vi "RFmx Analysis Only Configure Session.vi"(0 "IVI Refnum in":refnum<k15>="RFSA" caption="Resource Name", 1 "Span (Hz)":dbl=765000000.0 format="%.3p", 5 "Carrier Frequency (Hz)":dbl=4000000000.0 format="%#_6p", 7 "Reference Level (dBm)":dbl format="%.2f", 9 "number of records":i64=1, 11 "error in (no error)":errorcluster) -> (4 "RFSA Instrument Handle Out":refnum<k15>, 6 "RFmx Instrument Handle Out":T4, 15 "error out 2":errorcluster)   [LabVIEW 2017]
uses:
  <instrlib>/niRFSA/niRFSA.llb/niRFSA Ref Clock Sources.ctl
  <instrlib>/niRFSA/niRFSA.llb/niRFSA Exported Signal Destinations.ctl
  <instrlib>/niRFSA/niRFSA.llb/niRFSA Trigger Terminals.ctl
  <vilib>/RFmx/RFInstr/mx/Support/RFmxInstrSupport.llb/niRFmx Instrument Handle.ctl
  <instrlib>/niRFSA/niRFSA.llb/niRFSA Acquisition Types.ctl
  <instrlib>/niRFSA/niRFSA.llb/niRFSA Signal Names.ctl
  <vilib>/RFmx/SpecAn/mx/RFmxSpecAn.llb/RFmxSpecAn Select Measurement (Multiple).vi
  <instrlib>/niRFSA/niRFSA.llb/niRFSA Configure Digital Edge Start Trigger.vi
  <instrlib>/niRFSA/niRFSA.llb/niRFSA Configure Digital Edge Advance Trigger.vi
  <resource>/objmgr/RFmxInstr.rc
panel:
  in  "Integration Bandwidth (Hz)":dbl=5000000.0 format="%.3p"
  in  "source":T1="PXI_Trig0"
  in  "output terminal":T2="PXI_Trig1"
  in  "Clock Source":T3="OnboardClock"
  # "RFSA Settings"
  # "RFmx Settings"
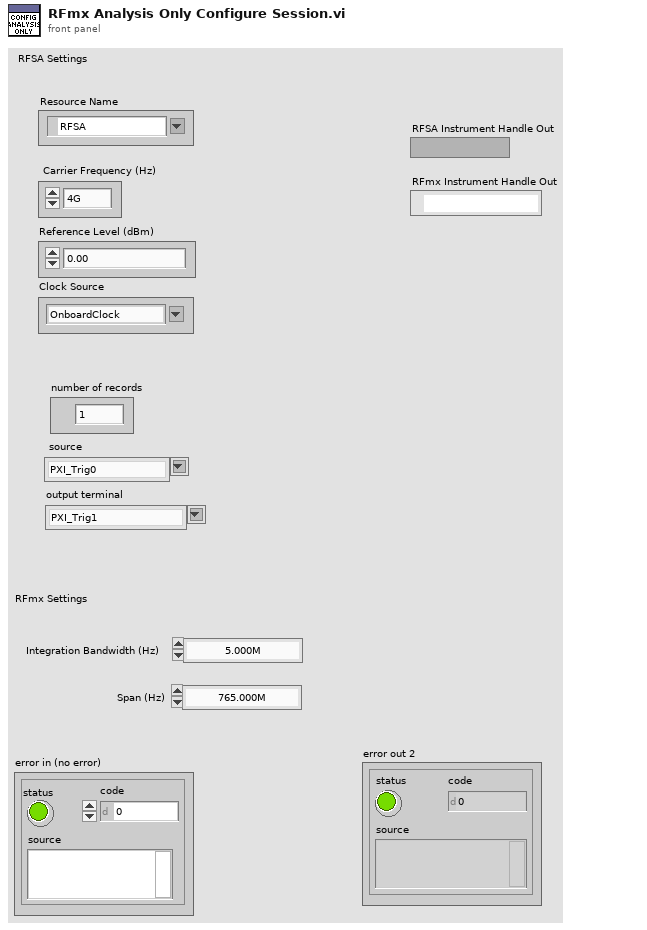
[diagram p1: front panel]
types:
  T1 = typedef "niRFSA Trigger Terminals.ctl" = string
  T2 = typedef "niRFSA Exported Signal Destinations.ctl" = string
  T3 = typedef "niRFSA Ref Clock Sources.ctl" = string
  T4 = typedef "niRFmx Instrument Handle.ctl" = refnum<k21>
  T5 = enum16{"ACP", "CCDF", "CHP", "FCnt", "Harmonics", "OBW", "SEM", "Spectrum", "Spur", "TXP", "AMPM", "DPD", "IQ", "IM", "NF", "PhaseNoise"}[]
  T6 = typedef "niRFSA Signal Names.ctl" = i32
  T7 = typedef "niRFSA Acquisition Types.ctl" = i32
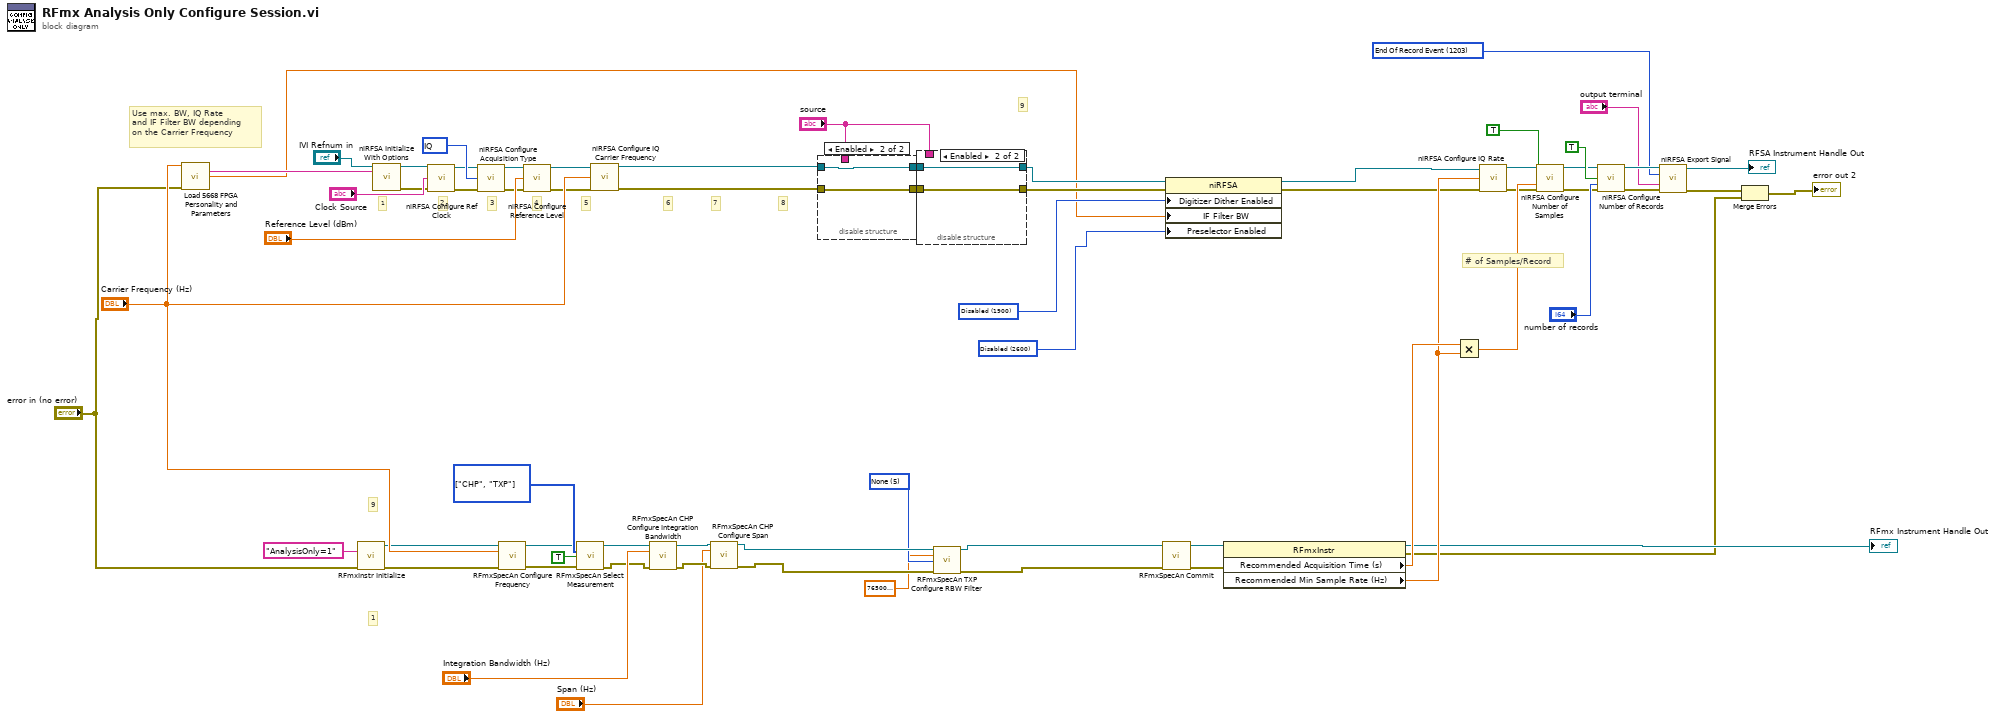
[diagram p0: block diagram]
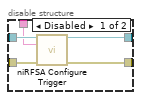
[diagram p2: hidden frame]
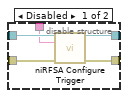
[diagram p3: hidden frame]
diagram:
  w3 = 5 items=["None"=5, "Gaussian"=1, "Flat"=2, "RRC"=6] ("RBW Filter Type")
  w67 = T5 [enum."CHP", enum."TXP"] items=["ACP", "CCDF", "CHP", "FCnt", "Harmonics", "OBW", "SEM", "Spectrum", "Spur", "TXP", "AMPM", "DPD", "IQ", "IM", "NF", "PhaseNoise"] ("Measurements")
  w45 = 2600 items=["Disabled"=2600, "Enabled when in Signal Path"=2601, "Enabled"=2602] ("Signal Path:Advanced:Downconverter Preselector Enabled")
  w44 = 1900 items=["Disabled"=1900, "Enabled"=1901] ("Signal Path:Digitizer Dither Enabled")
  w32 = T6 1203 items=["Start Trigger"=1100, "Ref Trigger"=702, "Advance Trigger"=1102, "Ready For Start Event"=1200, "Ready For Ref Event"=1201, "Ready For Advance Event"=1202, "End Of Record Event"=1203, "Done Event"=1204, "Reference Clock"=1205, "User"=1206] ("signal")
  w30 = T7 100 items=["IQ"=100, "Spectrum"=101] ("acquisition type")
  # "# of Samples/Record"
  # "Use max. BW, IQ Rate \nand IF Filter BW depending \non the Carrier Frequency"
  # "9"
  # "8"
  # "7"
  # "6"
  # "5"
  # "4"
  # "3"
  # "2"
  # "1"
  # "9"
  # "1"
  n1 = call "Load 5668 FPGA Personality and Parameters.vi"("Start Carrier Frequency in"="Carrier Frequency (Hz)", "error in"="error in (no error)") -> ("option string"=w46:string, "Signal Path:IF Filter Bandwidth"=w7:dbl)  [unwired: 9 in, 3 out]
  n2 = call <vilib>:"RFmxInstr Initialize.vi"("Option String"="AnalysisOnly=1", "error in (no error)"="error in (no error)") -> ("Instrument Handle Out"=w12:refnum<k21>, "error out"=w13:errorcluster)  [unwired: 11 in, 1 out]
  n3 = call <instrlib>:"niRFSA Initialize With Options.vi"("resource name"="IVI Refnum in", "option string"=w46) -> ("instrument handle out"=w22:refnum<k15>, "error out"=w23:errorcluster)  [unwired: 12 in]
  n4 = call <instrlib>:"niRFSA Configure Ref Clock.vi"("instrument handle"=w22, "clock source"="Clock Source", "error in"=w23) -> ("instrument handle out"=w27:refnum<k15>, "error out"=w26:errorcluster)  [unwired: 11 in]
  n5 = call <instrlib>:"niRFSA Configure Acquisition Type.vi"("instrument handle"=w27, "acquisition type"=w30, "error in"=w26) -> ("instrument handle out"=w24:refnum<k15>, "error out"=w25:errorcluster)  [unwired: 11 in]
  n6 = call <vilib>:"RFmxSpecAn Configure Frequency.vi"("Instrument Handle In"=w12, "Center Frequency (Hz)"="Carrier Frequency (Hz)", "error in (no error)"=w13) -> ("Instrument Handle Out"=w15:refnum<k21>, "error out"=w16:errorcluster)  [unwired: 11 in]
  n7 = call <instrlib>:"niRFSA Configure Reference Level.vi"("instrument handle"=w24, "reference level (dBm)"="Reference Level (dBm)", "error in"=w25) -> ("instrument handle out"=w34:refnum<k15>, "error out"=w36:errorcluster)  [unwired: 11 in]
  n8 = call-poly <vilib>:"RFmxSpecAn Select Measurement.vi"("Instrument Handle In"=w15, "Measurements"=w67, "Enable All Traces"=TRUE, "error in (no error)"=w16) -> ("Instrument Handle Out"=w17:refnum<k21>, "error out"=w18:errorcluster)  [unwired: 10 in]
  n9 = call <instrlib>:"niRFSA Configure IQ Carrier Frequency.vi"("instrument handle"=w34, "carrier frequency"="Carrier Frequency (Hz)", "error in"=w36) -> ("instrument handle out"=w35:refnum<k15>, "error out"=w37:errorcluster)  [unwired: 11 in]
  n10 = call <vilib>:"RFmxSpecAn CHP Configure Integration Bandwidth.vi"("Instrument Handle In"=w17, "Integration Bandwidth (Hz)"="Integration Bandwidth (Hz)", "error in (no error)"=w18) -> ("Instrument Handle Out"=w20:refnum<k21>, "error out"=w21:errorcluster)  [unwired: 11 in]
  n11 = call <vilib>:"RFmxSpecAn CHP Configure Span.vi"("Instrument Handle In"=w20, "Span (Hz)"="Span (Hz)", "error in (no error)"=w21) -> ("Instrument Handle Out"=w5:refnum<k21>, "error out"=w50:errorcluster)  [unwired: 11 in]
  n12 = disable-structure shown="Enabled" {
    disable-tunnel: w37 -> [w72 w73]
    disable-tunnel: [w71 w73] -> w39
    disable-tunnel: w35 -> [w70 w74]
    disable-tunnel: [w69 w74] -> w40
    disable-tunnel: "source" -> [w68 _]
    frame Disabled {
      n13 = call-poly <instrlib>:"niRFSA Configure Trigger.vi"("instrument handle"=w70, "source"=w68, "error in"=w72) -> ("instrument handle out"=w69:refnum<k15>, "error out"=w71:errorcluster)  [unwired: 11 in]
    }
    frame Enabled {
    }
  }
  n14 = disable-structure shown="Enabled" {
    disable-tunnel: [w79 w80] -> w38
    disable-tunnel: [w78 w81] -> w43
    disable-tunnel: w39 -> [w77 w80]
    disable-tunnel: w40 -> [w76 w81]
    disable-tunnel: "source" -> [w75 _]
    frame Disabled {
      n15 = call-poly <instrlib>:"niRFSA Configure Trigger.vi"("instrument handle"=w76, "source"=w75, "error in"=w77) -> ("instrument handle out"=w78:refnum<k15>, "error out"=w79:errorcluster)  [unwired: 11 in]
    }
    frame Enabled {
    }
  }
  n16 = call <vilib>:"RFmxSpecAn TXP Configure RBW Filter.vi"("Instrument Handle In"=w5, "RBW (Hz)"=765000000.0, "RBW Filter Type"=w3, "error in (no error)"=w50) -> ("Instrument Handle Out"=w4:refnum<k21>, "error out"=w6:errorcluster)  [unwired: 10 in]
  n17 = call <vilib>:"RFmxSpecAn Commit.vi"("Instrument Handle In"=w4, "error in (no error)"=w6) -> ("Instrument Handle Out"=w52:refnum<k21>, "error out"=w51:errorcluster)  [unwired: 12 in]
  n18 = property class="niRFSA"(reference=w43, error in=w38, "Digitizer Dither Enabled"=w44, "IF Filter BW"=w7, "Preselector Enabled"=w45) -> (reference out=w54:refnum<k15>, error out=w42:errorcluster)
  n19 = property class="RFmxInstr"(reference=w52, error in=w51) -> (reference out=→"RFmx Instrument Handle Out":refnum<k21>, error out=w9:errorcluster, "Recommended Acquisition Time (s)"=w58:dbl, "Recommended Min Sample Rate (Hz)"=w57:dbl)
  n20 = Multiply(x=w58, y=w57) -> (x*y=w66:dbl)
  n21 = call <instrlib>:"niRFSA Configure IQ Rate.vi"("instrument handle"=w54, "IQ rate (S/s)"=w57, "error in"=w42) -> ("instrument handle out"=w56:refnum<k15>, "error out"=w53:errorcluster)  [unwired: 11 in]
  n22 = call <instrlib>:"niRFSA Configure Number of Samples.vi"("instrument handle"=w56, "number of samples is finite"=TRUE, "samples per record"=w66, "error in"=w53) -> ("instrument handle out"=w62:refnum<k15>, "error out"=w55:errorcluster)  [unwired: 10 in]
  n23 = call <instrlib>:"niRFSA Configure Number of Records.vi"("instrument handle"=w62, "number of records is finite"=TRUE, "number of records"="number of records", "error in"=w55) -> ("instrument handle out"=w63:refnum<k15>, "error out"=w61:errorcluster)  [unwired: 10 in]
  n24 = call <instrlib>:"niRFSA Export Signal.vi"("instrument handle"=w63, "signal"=w32, "output terminal"="output terminal", "error in"=w61) -> ("instrument handle out"=→"RFSA Instrument Handle Out":refnum<k15>, "error out"=w48:errorcluster)  [unwired: 10 in]
  n25 = Merge Errors(w48, w9) -> (→"error out 2":errorcluster)
